vi "Generate waveform.vi"(8 "error in (no error)":errorcluster, 11 "Galvo in":refnum<class "InVivo_ImagingModeSPIM.lvclass">) -> (0 "error out":errorcluster, 2 "Array":variant[](array[variant]), 3 "Galvo out":refnum<class "InVivo_ImagingModeSPIM.lvclass">)   [LabVIEW 2012, in "InVivo_ImagingModeSPIM.lvclass"]
uses:
  InVivo_ImagingModeSPIM.lvclass
  InVivo_ImagingModeSPIM.lvclass/InVivo_ImagingModeSPIM.ctl
  <vilib>/measure/NI_MABase.lvlib
panel:
  out "Waveformvalues":variant
  out "Mixed Signal Graph 2":waveform(dbl)(graph)
  out "Mixed Signal Graph":waveform(dbl)[](graph)
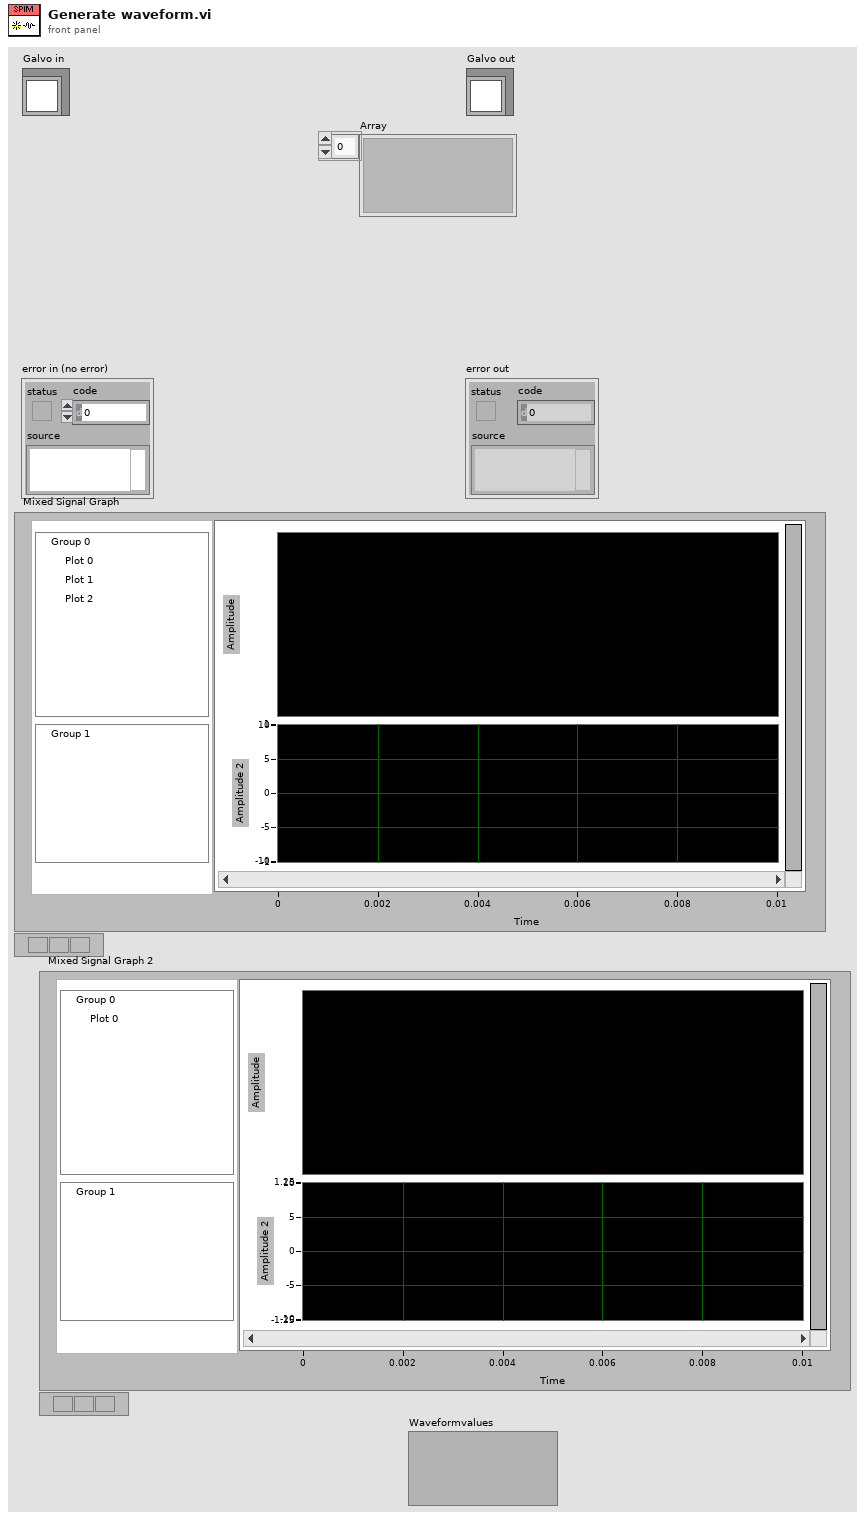
[diagram p1: front panel]
types:
  T1 = typedef "InVivo_ImagingModeSPIM.lvclass/waveform_enum.ctl" = enum16{"triangular", "sawtooth", "sinusodial"}
  T2 = typedef "InVivo_ImagingModeSPIM.lvclass/Control 4.ctl" = enum16{"Triangular", "Sawtooth", "Sinusoidal"}
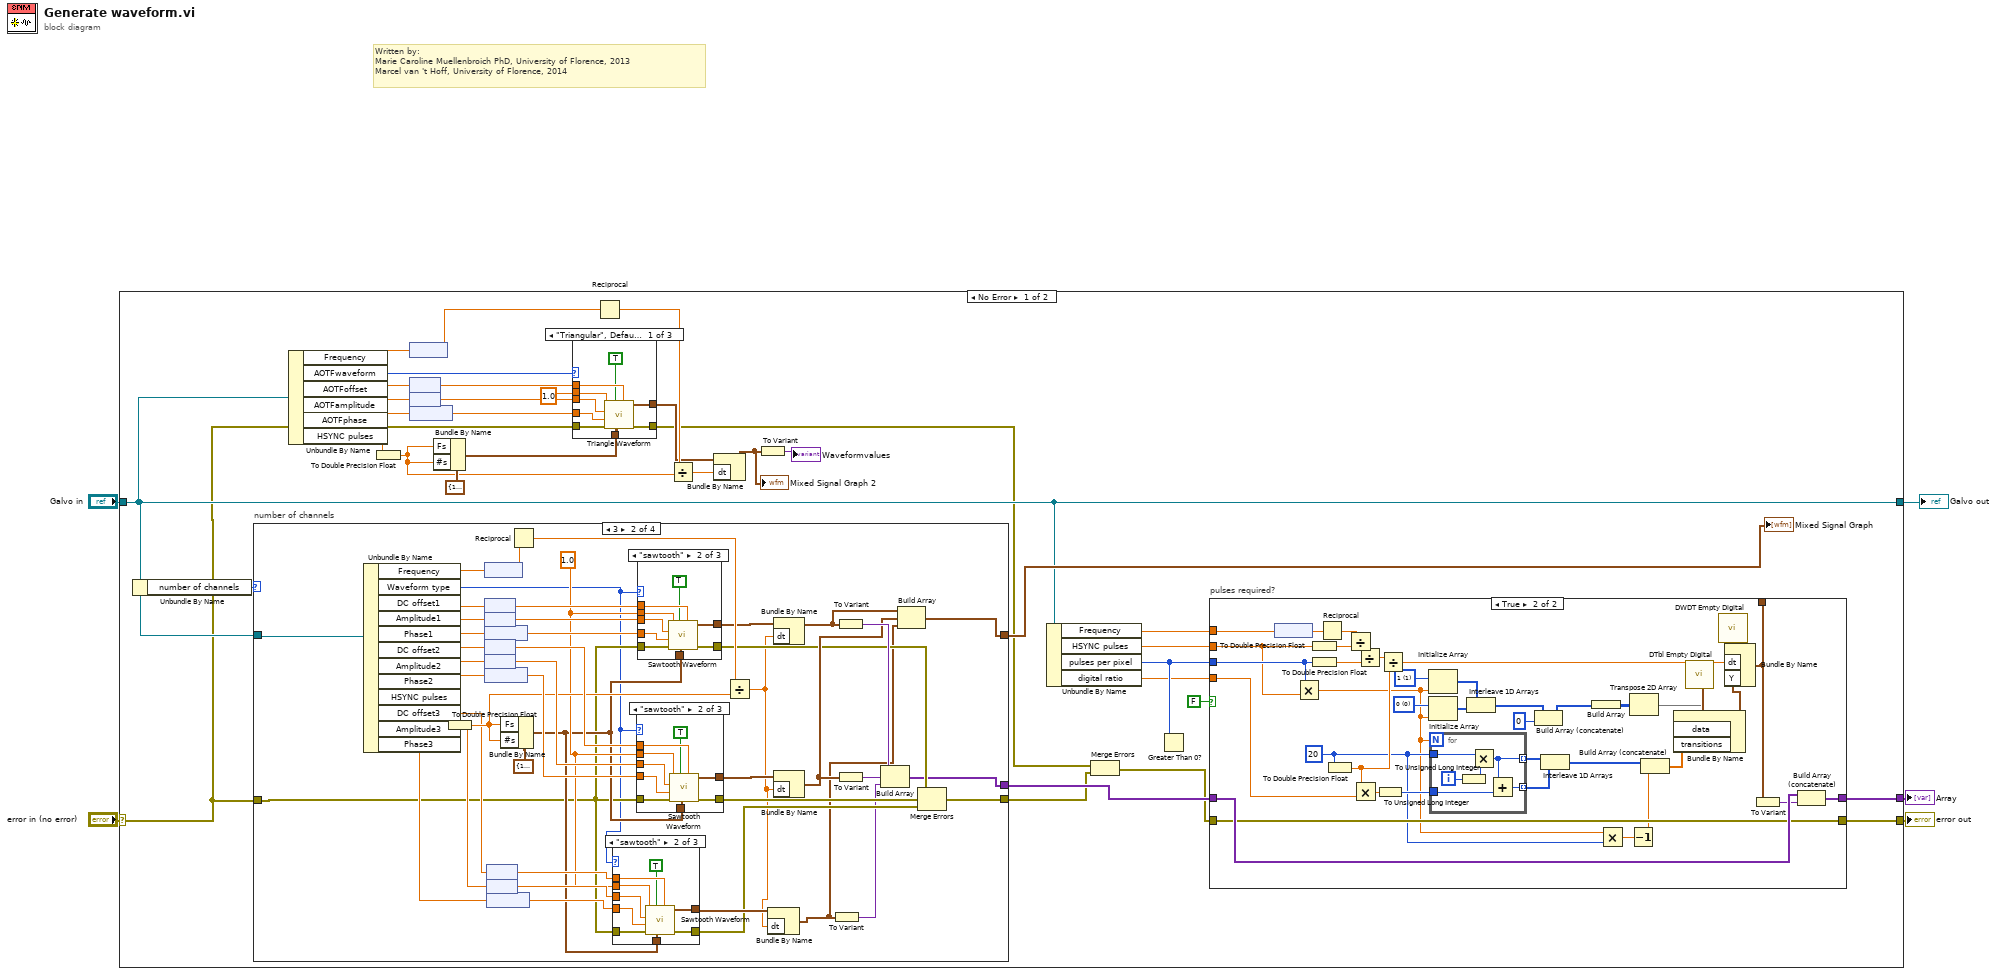
[diagram p0: block diagram]
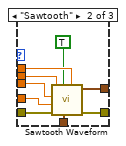
[diagram p2: hidden frame]
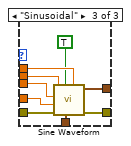
[diagram p3: hidden frame]
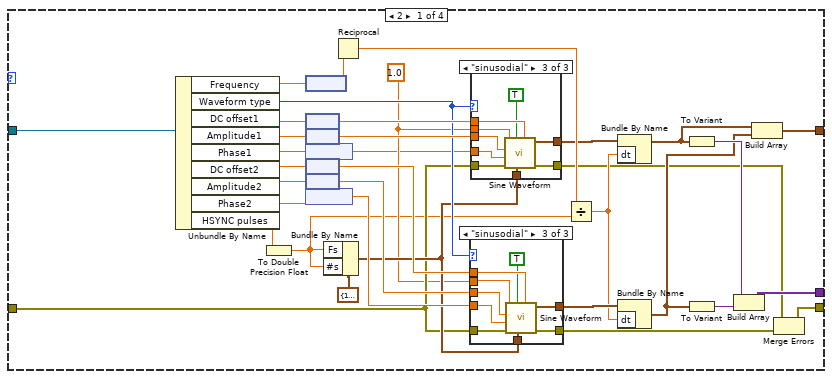
[diagram p5: hidden frame]
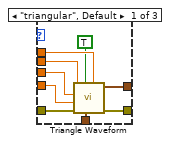
[diagram p6: hidden frame]
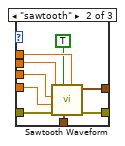
[diagram p7: hidden frame]
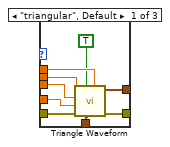
[diagram p8: hidden frame]
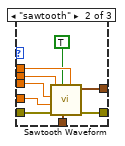
[diagram p9: hidden frame]
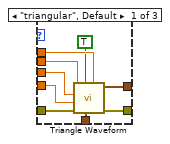
[diagram p10: hidden frame]
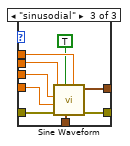
[diagram p11: hidden frame]
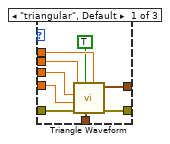
[diagram p12: hidden frame]
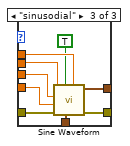
[diagram p13: hidden frame]
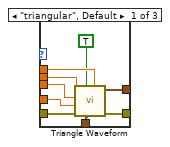
[diagram p14: hidden frame]
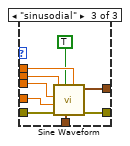
[diagram p15: hidden frame]
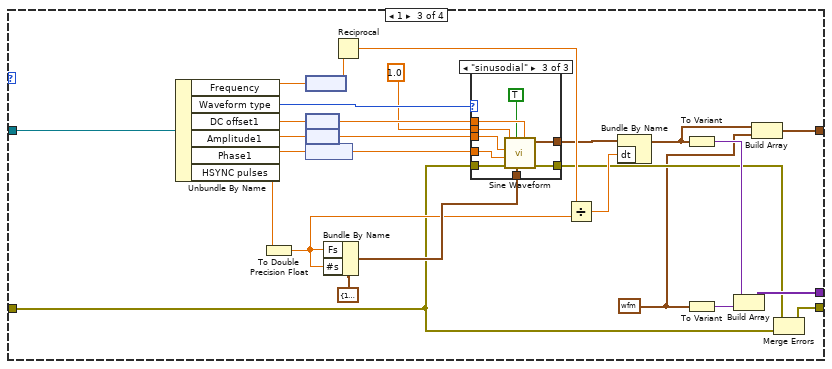
[diagram p16: hidden frame]
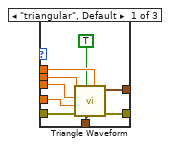
[diagram p17: hidden frame]
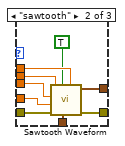
[diagram p18: hidden frame]
diagram:
  # "Written by:\nMarie Caroline Muellenbroich PhD, University of Florence, 2013 \nMarcel van 't Hoff, University of Florence, 2014"
  n1 = case shown="No Error" "error in (no error)" {
    selector: "error in (no error)" -> [w28 w385]
    tunnel: [w34 w385] -> w5
    tunnel: [w29 w384] -> w4
    tunnel: "Galvo in" -> [w29 w384]
    tunnel: [w39 _] -> w3
    frame No Error {
      n2 = Unbundle By Name(w29) -> ("number of channels"=w31:u8)
      n3 = case "number of channels" shown="3" w31 {
        tunnel: [w132 w208 w346 w383] -> w9
        tunnel: w28 -> [w133 w204 w331 w383]
        tunnel: [w131 w206 w345 _] -> w38
        tunnel: [w117 w207 w334 _] -> w30
        tunnel: w29 -> [w114 w205 w329 _]
        frame 2 {
          w127 = 1.0
          n4 = Unbundle By Name(w114) -> ("Frequency"=w124:dbl[unit], "Waveform type"=w142:T1, "DC offset1"=w143:dbl[unit], "Amplitude1"=w144:dbl[unit], "Phase1"=w145:dbl[unit], "DC offset2"=w140:dbl[unit], "Amplitude2"=w139:dbl[unit], "Phase2"=w138:dbl[unit], "HSYNC pulses"=w137:dbl)
          n5 = To Double Precision Float(number=w137) -> (double precision float=w122:dbl)
          n6 = node(w124) -> (w126:dbl)
          n7 = node(w143) -> (w147:dbl)
          n8 = node(w144) -> (w148:dbl)
          n9 = node(w145) -> (w123:dbl)
          n10 = node(w140) -> (w141:dbl)
          n11 = node(w139) -> (w135:dbl)
          n12 = node(w138) -> (w136:dbl)
          n13 = Bundle By Name(cluster=cluster{"Fs":dbl, "#s":dbl} {"Fs"=1000.0, "#s"=1000.0} ("sampling info"), "Fs"=w122, "#s"=w122) -> (w134:cluster{"Fs":dbl, "#s":dbl})
          n14 = Reciprocal(x=w126) -> (1/x=w121:dbl)
          n15 = case shown="\"sinusodial\"" w142 {
            tunnel: w141 -> [w155 w166 w175]
            tunnel: w127 -> [w154 w165 w174]
            tunnel: w134 -> [w156 w164 w173]
            tunnel: [w153 w163 w172] -> w125
            tunnel: [w157 w158 w167] -> w128
            tunnel: w135 -> [w150 w161 w170]
            tunnel: w136 -> [w151 w160 w169]
            tunnel: w133 -> [w149 w159 w168]
            frame "triangular", Default {
              n16 = call <vilib>:"Triangle Waveform.vi"("offset"=w155, "sampling info"=w156, "reset signal"=TRUE, "error in (no error)"=w149, "phase"=w151, "amplitude"=w150, "frequency"=w154) -> ("error out"=w157:errorcluster, "signal out"=w153:waveform(dbl))  [unwired: 3 in]
            }
            frame "sawtooth" {
              n17 = call <vilib>:"Sawtooth Waveform.vi"("offset"=w166, "sampling info"=w164, "reset signal"=TRUE, "error in (no error)"=w159, "phase"=w160, "amplitude"=w161, "frequency"=w165) -> ("error out"=w158:errorcluster, "signal out"=w163:waveform(dbl))  [unwired: 3 in]
            }
            frame "sinusodial" {
              n18 = call <vilib>:"Sine Waveform.vi"("offset"=w175, "sampling info"=w173, "reset signal"=TRUE, "error in (no error)"=w168, "phase"=w169, "amplitude"=w170, "frequency"=w174) -> ("error out"=w167:errorcluster, "signal out"=w172:waveform(dbl))  [unwired: 3 in]
            }
          }
          n19 = case shown="\"sinusodial\"" w142 {
            tunnel: w147 -> [w182 w193 w202]
            tunnel: w127 -> [w181 w192 w201]
            tunnel: w148 -> [w180 w191 w200]
            tunnel: w123 -> [w179 w190 w199]
            tunnel: w134 -> [w183 w189 w198]
            tunnel: [w178 w188 w197] -> w118
            tunnel: [w184 w187 w196] -> w115
            tunnel: w133 -> [w176 w185 w194]
            frame "triangular", Default {
              n20 = call <vilib>:"Triangle Waveform.vi"("offset"=w182, "sampling info"=w183, "reset signal"=TRUE, "error in (no error)"=w176, "phase"=w179, "amplitude"=w180, "frequency"=w181) -> ("error out"=w184:errorcluster, "signal out"=w178:waveform(dbl))  [unwired: 3 in]
            }
            frame "sawtooth" {
              n21 = call <vilib>:"Sawtooth Waveform.vi"("offset"=w193, "sampling info"=w189, "reset signal"=TRUE, "error in (no error)"=w185, "phase"=w190, "amplitude"=w191, "frequency"=w192) -> ("error out"=w187:errorcluster, "signal out"=w188:waveform(dbl))  [unwired: 3 in]
            }
            frame "sinusodial" {
              n22 = call <vilib>:"Sine Waveform.vi"("offset"=w202, "sampling info"=w198, "reset signal"=TRUE, "error in (no error)"=w194, "phase"=w199, "amplitude"=w200, "frequency"=w201) -> ("error out"=w196:errorcluster, "signal out"=w197:waveform(dbl))  [unwired: 3 in]
            }
          }
          n23 = Divide(x=w121, y=w122) -> (x/y=w120:dbl)
          n24 = Bundle By Name(cluster=w118, "dt"=w120) -> (w116:waveform(dbl))
          n25 = Bundle By Name(cluster=w125, "dt"=w120) -> (w119:waveform(dbl))
          n26 = To Variant(anything=w116) -> (Variant=w129:variant)
          n27 = To Variant(anything=w119) -> (Variant=w130:variant)
          n28 = Build Array(w129, w130) -> (w131:variant[])
          n29 = Build Array(w116, w119) -> (w117:waveform(dbl)[])
          n30 = Merge Errors(w115, w128) -> (w132:errorcluster)
        }
        frame 3 {
          w215 = 1.0
          n31 = Unbundle By Name(w205) -> ("Frequency"=w229:dbl[unit], "Waveform type"=w203:T1, "DC offset1"=w242:dbl[unit], "Amplitude1"=w243:dbl[unit], "Phase1"=w244:dbl[unit], "DC offset2"=w240:dbl[unit], "Amplitude2"=w239:dbl[unit], "Phase2"=w238:dbl[unit], "HSYNC pulses"=w237:dbl, "DC offset3"=w221:dbl[unit], "Amplitude3"=w220:dbl[unit], "Phase3"=w219:dbl[unit])
          n32 = To Double Precision Float(number=w237) -> (double precision float=w227:dbl)
          n33 = node(w229) -> (w231:dbl)
          n34 = node(w242) -> (w246:dbl)
          n35 = node(w243) -> (w247:dbl)
          n36 = node(w244) -> (w228:dbl)
          n37 = node(w240) -> (w241:dbl)
          n38 = node(w239) -> (w235:dbl)
          n39 = node(w238) -> (w236:dbl)
          n40 = node(w221) -> (w218:dbl)
          n41 = node(w220) -> (w217:dbl)
          n42 = node(w219) -> (w216:dbl)
          n43 = Bundle By Name(cluster=cluster{"Fs":dbl, "#s":dbl} {"Fs"=1000.0, "#s"=1000.0} ("sampling info"), "Fs"=w227, "#s"=w227) -> (w214:cluster{"Fs":dbl, "#s":dbl})
          n44 = Reciprocal(x=w231) -> (1/x=w226:dbl)
          n45 = case shown="\"sawtooth\"" w203 {
            tunnel: w218 -> [w254 w265 w274]
            tunnel: w215 -> [w253 w264 w273]
            tunnel: w214 -> [w255 w263 w272]
            tunnel: [w252 w262 w271] -> w213
            tunnel: [w256 w257 w266] -> w212
            tunnel: w217 -> [w249 w260 w269]
            tunnel: w216 -> [w250 w259 w268]
            tunnel: w204 -> [w248 w258 w267]
            frame "triangular", Default {
              n46 = call <vilib>:"Triangle Waveform.vi"("offset"=w254, "sampling info"=w255, "reset signal"=TRUE, "error in (no error)"=w248, "phase"=w250, "amplitude"=w249, "frequency"=w253) -> ("error out"=w256:errorcluster, "signal out"=w252:waveform(dbl))  [unwired: 3 in]
            }
            frame "sawtooth" {
              n47 = call <vilib>:"Sawtooth Waveform.vi"("offset"=w265, "sampling info"=w263, "reset signal"=TRUE, "error in (no error)"=w258, "phase"=w259, "amplitude"=w260, "frequency"=w264) -> ("error out"=w257:errorcluster, "signal out"=w262:waveform(dbl))  [unwired: 3 in]
            }
            frame "sinusodial" {
              n48 = call <vilib>:"Sine Waveform.vi"("offset"=w274, "sampling info"=w272, "reset signal"=TRUE, "error in (no error)"=w267, "phase"=w268, "amplitude"=w269, "frequency"=w273) -> ("error out"=w266:errorcluster, "signal out"=w271:waveform(dbl))  [unwired: 3 in]
            }
          }
          n49 = case shown="\"sawtooth\"" w203 {
            tunnel: w241 -> [w281 w292 w301]
            tunnel: w215 -> [w280 w291 w300]
            tunnel: w214 -> [w282 w290 w299]
            tunnel: [w279 w289 w298] -> w230
            tunnel: [w283 w284 w293] -> w232
            tunnel: w235 -> [w276 w287 w296]
            tunnel: w236 -> [w277 w286 w295]
            tunnel: w204 -> [w275 w285 w294]
            frame "triangular", Default {
              n50 = call <vilib>:"Triangle Waveform.vi"("offset"=w281, "sampling info"=w282, "reset signal"=TRUE, "error in (no error)"=w275, "phase"=w277, "amplitude"=w276, "frequency"=w280) -> ("error out"=w283:errorcluster, "signal out"=w279:waveform(dbl))  [unwired: 3 in]
            }
            frame "sawtooth" {
              n51 = call <vilib>:"Sawtooth Waveform.vi"("offset"=w292, "sampling info"=w290, "reset signal"=TRUE, "error in (no error)"=w285, "phase"=w286, "amplitude"=w287, "frequency"=w291) -> ("error out"=w284:errorcluster, "signal out"=w289:waveform(dbl))  [unwired: 3 in]
            }
            frame "sinusodial" {
              n52 = call <vilib>:"Sine Waveform.vi"("offset"=w301, "sampling info"=w299, "reset signal"=TRUE, "error in (no error)"=w294, "phase"=w295, "amplitude"=w296, "frequency"=w300) -> ("error out"=w293:errorcluster, "signal out"=w298:waveform(dbl))  [unwired: 3 in]
            }
          }
          n53 = case shown="\"sawtooth\"" w203 {
            tunnel: w246 -> [w308 w319 w328]
            tunnel: w215 -> [w307 w318 w327]
            tunnel: w247 -> [w306 w317 w326]
            tunnel: w228 -> [w305 w316 w325]
            tunnel: w214 -> [w309 w315 w324]
            tunnel: [w304 w314 w323] -> w224
            tunnel: [w310 w313 w322] -> w222
            tunnel: w204 -> [w302 w311 w320]
            frame "triangular", Default {
              n54 = call <vilib>:"Triangle Waveform.vi"("offset"=w308, "sampling info"=w309, "reset signal"=TRUE, "error in (no error)"=w302, "phase"=w305, "amplitude"=w306, "frequency"=w307) -> ("error out"=w310:errorcluster, "signal out"=w304:waveform(dbl))  [unwired: 3 in]
            }
            frame "sawtooth" {
              n55 = call <vilib>:"Sawtooth Waveform.vi"("offset"=w319, "sampling info"=w315, "reset signal"=TRUE, "error in (no error)"=w311, "phase"=w316, "amplitude"=w317, "frequency"=w318) -> ("error out"=w313:errorcluster, "signal out"=w314:waveform(dbl))  [unwired: 3 in]
            }
            frame "sinusodial" {
              n56 = call <vilib>:"Sine Waveform.vi"("offset"=w328, "sampling info"=w324, "reset signal"=TRUE, "error in (no error)"=w320, "phase"=w325, "amplitude"=w326, "frequency"=w327) -> ("error out"=w322:errorcluster, "signal out"=w323:waveform(dbl))  [unwired: 3 in]
            }
          }
          n57 = Divide(x=w226, y=w227) -> (x/y=w211:dbl)
          n58 = Bundle By Name(cluster=w213, "dt"=w211) -> (w209:waveform(dbl))
          n59 = Bundle By Name(cluster=w224, "dt"=w211) -> (w223:waveform(dbl))
          n60 = Bundle By Name(cluster=w230, "dt"=w211) -> (w225:waveform(dbl))
          n61 = To Variant(anything=w209) -> (Variant=w210:variant)
          n62 = To Variant(anything=w223) -> (Variant=w233:variant)
          n63 = To Variant(anything=w225) -> (Variant=w234:variant)
          n64 = Build Array(w233, w234, w210) -> (w206:variant[])
          n65 = Build Array(w223, w225, w209) -> (w207:waveform(dbl)[])
          n66 = Merge Errors(w222, w232, w212) -> (w208:errorcluster)
        }
        frame 1 {
          w330 = waveform(dbl) {"t0"=timestamp(0 s since 1904-01-01), "dt"=1.0, "Y"=[]} ("signal out")
          n67 = Unbundle By Name(w329) -> ("Frequency"=w340:dbl[unit], "Waveform type"=w349:T1, "DC offset1"=w350:dbl[unit], "Amplitude1"=w351:dbl[unit], "Phase1"=w352:dbl[unit], "HSYNC pulses"=w348:dbl)
          n68 = To Double Precision Float(number=w348) -> (double precision float=w338:dbl)
          n69 = node(w340) -> (w341:dbl)
          n70 = node(w350) -> (w354:dbl)
          n71 = node(w351) -> (w355:dbl)
          n72 = node(w352) -> (w339:dbl)
          n73 = Bundle By Name(cluster=cluster{"Fs":dbl, "#s":dbl} {"Fs"=1000.0, "#s"=1000.0} ("sampling info"), "Fs"=w338, "#s"=w338) -> (w347:cluster{"Fs":dbl, "#s":dbl})
          n74 = Reciprocal(x=w341) -> (1/x=w337:dbl)
          n75 = case shown="\"sinusodial\"" w349 {
            tunnel: w354 -> [w362 w373 w382]
            tunnel: 1.0 -> [w361 w372 w381]
            tunnel: w355 -> [w360 w371 w380]
            tunnel: w339 -> [w359 w370 w379]
            tunnel: w347 -> [w363 w369 w378]
            tunnel: [w358 w368 w377] -> w335
            tunnel: [w364 w367 w376] -> w332
            tunnel: w331 -> [w356 w365 w374]
            frame "triangular", Default {
              n76 = call <vilib>:"Triangle Waveform.vi"("offset"=w362, "sampling info"=w363, "reset signal"=TRUE, "error in (no error)"=w356, "phase"=w359, "amplitude"=w360, "frequency"=w361) -> ("error out"=w364:errorcluster, "signal out"=w358:waveform(dbl))  [unwired: 3 in]
            }
            frame "sawtooth" {
              n77 = call <vilib>:"Sawtooth Waveform.vi"("offset"=w373, "sampling info"=w369, "reset signal"=TRUE, "error in (no error)"=w365, "phase"=w370, "amplitude"=w371, "frequency"=w372) -> ("error out"=w367:errorcluster, "signal out"=w368:waveform(dbl))  [unwired: 3 in]
            }
            frame "sinusodial" {
              n78 = call <vilib>:"Sine Waveform.vi"("offset"=w382, "sampling info"=w378, "reset signal"=TRUE, "error in (no error)"=w374, "phase"=w379, "amplitude"=w380, "frequency"=w381) -> ("error out"=w376:errorcluster, "signal out"=w377:waveform(dbl))  [unwired: 3 in]
            }
          }
          n79 = Divide(x=w337, y=w338) -> (x/y=w336:dbl)
          n80 = Bundle By Name(cluster=w335, "dt"=w336) -> (w333:waveform(dbl))
          n81 = To Variant(anything=w333) -> (Variant=w343:variant)
          n82 = To Variant(anything=w330) -> (Variant=w344:variant)
          n83 = Build Array(w343, w344) -> (w345:variant[])
          n84 = Build Array(w333, w330) -> (w334:waveform(dbl)[])
          n85 = Merge Errors(w332, w331) -> (w346:errorcluster)
        }
        frame Default {
        }
      }
      "Mixed Signal Graph" <- w30
      n86 = Unbundle By Name(w29) -> ("Frequency"=w15:dbl[unit], "AOTFwaveform"=w20:T2, "AOTFoffset"=w21:dbl[unit], "AOTFamplitude"=w22:dbl[unit], "AOTFphase"=w23:dbl[unit], "HSYNC pulses"=w19:dbl)
      n87 = To Double Precision Float(number=w19) -> (double precision float=w13:dbl)
      n88 = node(w15) -> (w16:dbl)
      n89 = node(w21) -> (w25:dbl)
      n90 = node(w22) -> (w26:dbl)
      n91 = node(w23) -> (w14:dbl)
      n92 = Bundle By Name(cluster=cluster{"Fs":dbl, "#s":dbl} {"Fs"=1000.0, "#s"=1000.0} ("sampling info"), "Fs"=w13, "#s"=w13) -> (w18:cluster{"Fs":dbl, "#s":dbl})
      n93 = case shown="\"Triangular\", Default" w20 {
        tunnel: w25 -> [w46 w57 w66]
        tunnel: 1.0 -> [w45 w56 w65]
        tunnel: w26 -> [w44 w55 w64]
        tunnel: w14 -> [w43 w54 w63]
        tunnel: w18 -> [w47 w53 w62]
        tunnel: [w42 w52 w61] -> w10
        tunnel: [w48 w51 w60] -> w7
        tunnel: w28 -> [w40 w49 w58]
        frame "Triangular", Default {
          n94 = call <vilib>:"Triangle Waveform.vi"("offset"=w46, "sampling info"=w47, "reset signal"=TRUE, "error in (no error)"=w40, "phase"=w43, "amplitude"=w44, "frequency"=w45) -> ("error out"=w48:errorcluster, "signal out"=w42:waveform(dbl))  [unwired: 3 in]
        }
        frame "Sawtooth" {
          n95 = call <vilib>:"Sawtooth Waveform.vi"("offset"=w57, "sampling info"=w53, "reset signal"=TRUE, "error in (no error)"=w49, "phase"=w54, "amplitude"=w55, "frequency"=w56) -> ("error out"=w51:errorcluster, "signal out"=w52:waveform(dbl))  [unwired: 3 in]
        }
        frame "Sinusoidal" {
          n96 = call <vilib>:"Sine Waveform.vi"("offset"=w66, "sampling info"=w62, "reset signal"=TRUE, "error in (no error)"=w58, "phase"=w63, "amplitude"=w64, "frequency"=w65) -> ("error out"=w60:errorcluster, "signal out"=w61:waveform(dbl))  [unwired: 3 in]
        }
      }
      n97 = Reciprocal(x=w16) -> (1/x=w12:dbl)
      n98 = Divide(x=w12, y=w13) -> (x/y=w11:dbl)
      n99 = Bundle By Name(cluster=w10, "dt"=w11) -> (w6:waveform(dbl))
      "Mixed Signal Graph 2" <- w6
      n100 = To Variant(anything=w6) -> (Variant=→"Waveformvalues":variant)
      n101 = Unbundle By Name(w29) -> ("Frequency"=w37:dbl[unit], "HSYNC pulses"=w36:dbl, "pulses per pixel"=w35:i32, "digital ratio"=w33:dbl)
      n102 = Merge Errors(w7, w9) -> (w8:errorcluster)
      n103 = Greater Than 0?(x=w35) -> ()  [unwired: 1 out]
      n104 = case "pulses required?" shown="True" FALSE {
        tunnel: w35 -> [_ w72]
        tunnel: [w68 w89] -> w34
        tunnel: w8 -> [w68 w89]
        tunnel: [w67 w102] -> w39
        tunnel: w38 -> [w67 w103]
        tunnel: w37 -> [_ w107]
        tunnel: w36 -> [_ w69]
        tunnel: [_ w99] -> _
        tunnel: w33 -> [_ w85]
        frame False {
        }
        frame True {
          w73 = u32 20 ("ratio step size")
          w91 = u8 0 items=["0", "1", "Z", "L", "H", "X", "T", "V"] ("value 2")
          w90 = u8 1 items=["0", "1", "Z", "L", "H", "X", "T", "V"] ("value 2")
          n105 = node(w107) -> (w106:dbl)
          n106 = Multiply(x=w72, y=w69) -> (x*y=w70:dbl)
          n107 = To Double Precision Float(number=w69) -> (double precision float=w104:dbl)
          n108 = To Double Precision Float(number=w72) -> (double precision float=w100:dbl)
          n109 = Reciprocal(x=w106) -> (1/x=w105:dbl)
          n110 = To Double Precision Float(number=w73) -> (double precision float=w84:dbl)
          n111 = Divide(x=w105, y=w104) -> (x/y=w101:dbl)
          n112 = Multiply(x=w84, y=w85) -> (x*y=w95:dbl)
          n113 = Divide(x=w101, y=w100) -> (x/y=w83:dbl)
          n114 = To Unsigned Long Integer(number=w95) -> (unsigned 32bit integer=w98:u32)
          n115 = Divide(x=w83, y=w84) -> (x/y=w82:dbl)
          n116 = Initialize Array(w90, w70) -> (w93:u8[])
          n117 = Initialize Array(w91, w70) -> (w94:u8[])
          n118 = for {
            N: w70 -> [_]
            tunnel: w98 -> [w111]
            tunnel: w73 -> [w113]
            tunnel: [w110] -> w96 mode=indexing
            tunnel: [w109] -> w97 mode=indexing
            i -> [w112]
            n119 = To Unsigned Long Integer(number=w112) -> (unsigned 32bit integer=w108:u32)
            n120 = Multiply(x=w113, y=w108) -> (x*y=w110:u32)
            n121 = Add(x=w110, y=w111) -> (x+y=w109:u32)
          }
          n122 = Interleave 1D Arrays(w93, w94) -> (w78:u8[])
          n123 = Build Array (concatenate)(w78, u8 0 ("value 2")) -> (w77:u8[])
          n124 = Interleave 1D Arrays(w96, w97) -> (w76:u32[])
          n125 = Build Array(w77) -> (w92:u8[][])
          n126 = Multiply(x=w70, y=w73) -> (x*y=w74:dbl)
          n127 = Decrement(x=w74) -> (x-1=w71:dbl)
          n128 = Transpose 2D Array(2D array=w92) -> (transposed array=w80:u8[][])
          n129 = Build Array (concatenate)(w76, w71) -> (w75:dbl[])
          n130 = call <vilib>:"DTbl Empty Digital.vi"() -> ("digital data"=w88:digitaldata)  [unwired: 5 in]
          n131 = Bundle By Name(cluster=w88, "data"=w80, "transitions"=w75) -> (w86:digitaldata)
          n132 = call <vilib>:"DWDT Empty Digital.vi"() -> ("digital waveform out"=w87:digitalwaveform)  [unwired: 5 in]
          n133 = Bundle By Name(cluster=w87, "dt"=w82, "Y"=w86) -> (w99:digitalwaveform)
          n134 = To Variant(anything=w99) -> (Variant=w81:variant)
          n135 = Build Array (concatenate)(w103, w81) -> (w102:variant[])
        }
      }
    }
    frame Error {
    }
  }
  "error out" <- w5
  "Galvo out" <- w4
  "Array" <- w3
